vi "Configure DRAM Manager.vi"(0 "fpga interface in":refnum<k20>, 5 "serial output channels":string[](array[string]), 7 "elements per dram bank":u32, 9 "dram arbiter config":T1={"write grant time (clocks)"=1000, "read grant time (clocks)"=1000}, 11 "error in (no error)":errorcluster, 12 "write time slice":u16=500, 13 "request time slice":u16=500) -> (4 "fpga interface out":refnum<k20>, 6 "dram partition sizes (bytes)":u64[](array[numeric]), 15 "error out":errorcluster)   [LabVIEW 2023, in "GettingStarted_Gen_148X_Host.lvlib"]
uses:
  GettingStarted_Gen_148X_Host.lvlib
  Types/148x_Gen_FPGA_Reference.ctl
  <vilib>/Utility/error.llb/Error Cluster From Error Code.vi
  <vilib>/rvi/errors/niLvFpgaAdjustHostInterfaceError.vi
  <vilib>/rvi/interface/nirviReadWriteControl/nirviReadWriteControl.xnode
  <vilib>/rvi/interface/Simulation/niFpgaSimulationCallBeginRW.vi
  NiFpgaLv.dll
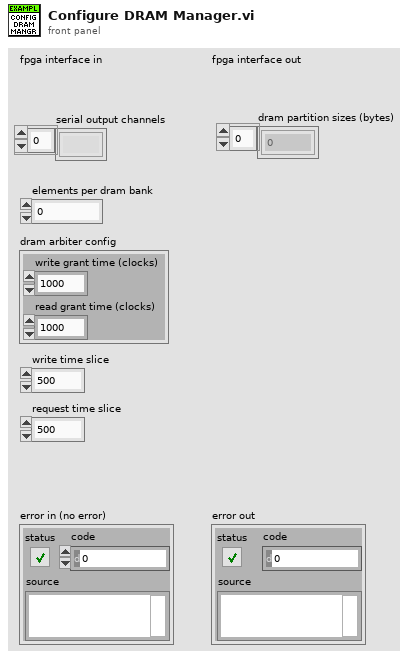
[diagram p1: front panel]
types:
  T1 = cluster{"write grant time (clocks)":u16, "read grant time (clocks)":u16}
  T2 = typedef "GettingStarted_Gen_148X_Host.lvlib/148x_Gen_FPGA_Reference.ctl" = refnum<k20>
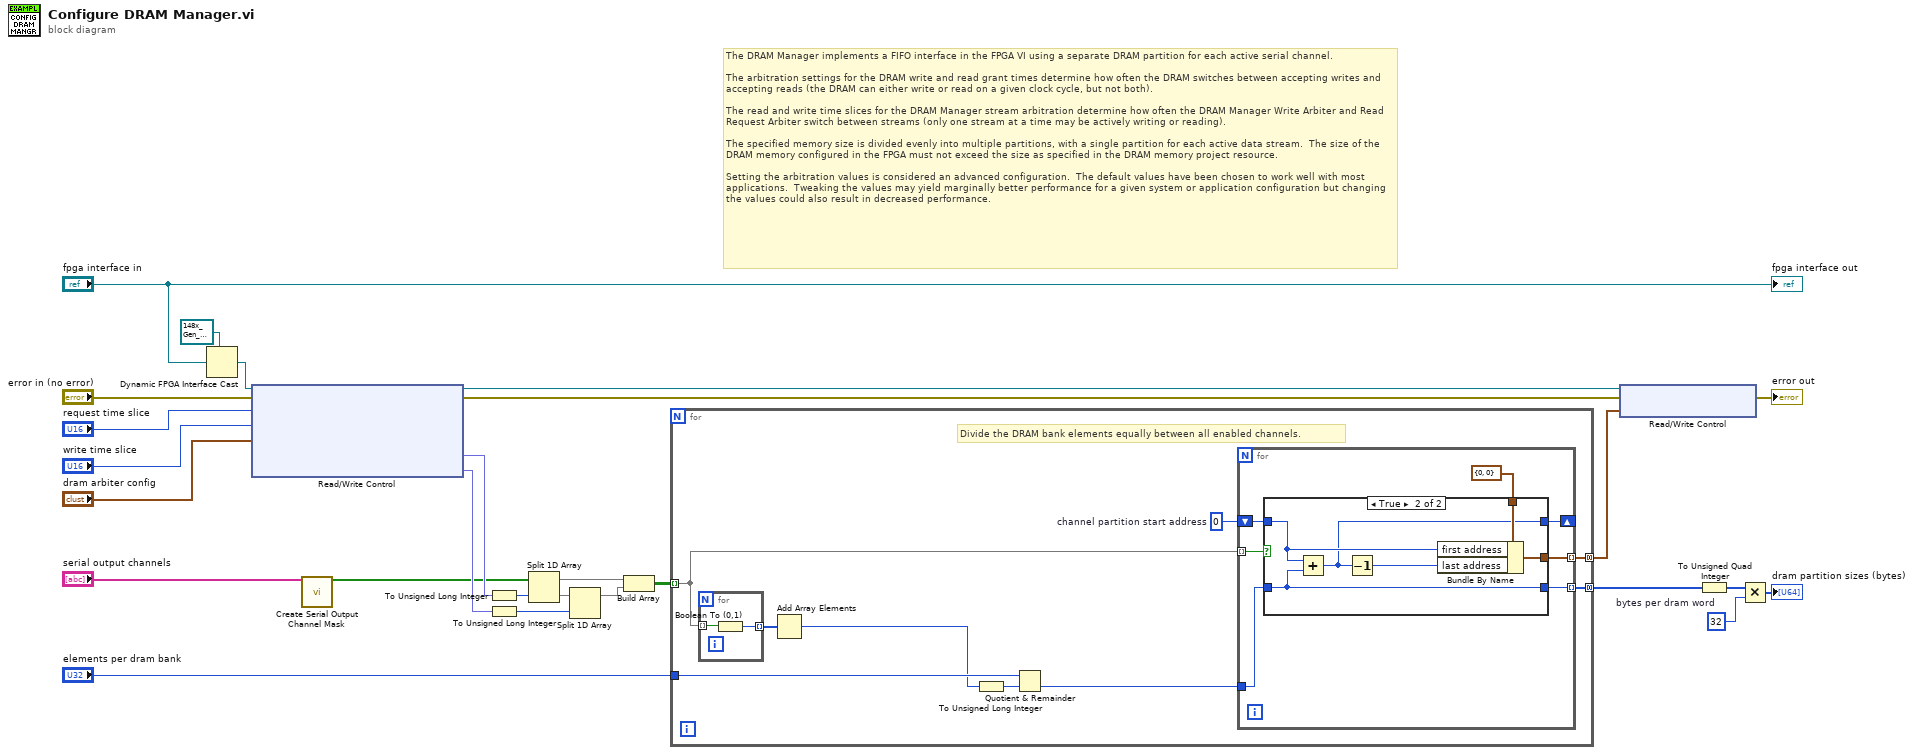
[diagram p0: block diagram]
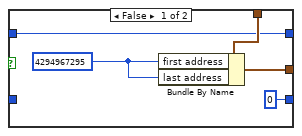
[diagram p2: hidden frame]
diagram:
  w4 = u64 32  # bytes per dram word
  # "The DRAM Manager implements a FIFO interface in the FPGA VI using a separate DRAM partition for each active serial channel.  \n\nThe arbitration settings for the DRAM write and read grant times determine how often the DRAM switches between accepting writes and accepting reads (the DRAM can either write or read on a given clock cycle, but not both).  \n\nThe read and write time slices for the DRAM Manager stream arbitration determine how often the DRAM Manager Write Arbiter and Read Request Arbiter switch between streams (only one stream at a time may be actively writing or reading).  \n\nThe specified memory size is divided evenly into multiple partitions, with a single partition for each active data stream.  The size of the DRAM memory configured in the FPGA must not exceed the size as specified in the DRAM memory project resource.  \n\nSetting the arbitration values is considered an advanced configuration.  The default values have been chosen to work well with most applications.  Tweaking the values may yield marginally better performance for a given system or application configuration but changing the values could also result in decreased performance."
  n1 = Dynamic FPGA Interface Cast(Session In=T2 refnum ("FPGA VI Reference Out"), Type="fpga interface in") -> (Session Out=w14:T2)
  n2 = xnode "Read/Write Control"("FPGA VI Reference In"=w14, "error in"="error in (no error)", "request time slice"="request time slice", "write time slice"="write time slice", "dram arbiter config"="dram arbiter config") -> ("FPGA VI Reference Out"=w22:T2, "error out"=w20:errorcluster, "dram manager 0.num active streams"=w19:fxp<+,3,3>, "dram manager 1.num active streams"=w8:fxp<+,3,3>)
  n3 = call "Create Serial Output Channel Mask.vi"("serial channels"="serial output channels") -> ("serial output channel mask"=w7:bool[])  [unwired: 14 in]
  n4 = To Unsigned Long Integer(number=w19) -> (unsigned 32bit integer=w10:u32)
  n5 = To Unsigned Long Integer(number=w8) -> (unsigned 32bit integer=w9:u32)
  n6 = Split 1D Array(array=w7, index=w10) -> (first subarray=w24:bool[], second subarray=w12:bool[])
  n7 = Split 1D Array(array=w12, index=w9) -> (first subarray=w11:bool[])  [unwired: 1 out]
  n8 = Build Array(w24, w11) -> (w23:bool[][])
  n9 = for {
    tunnel: "elements per dram bank" -> [w35]
    tunnel: w23 -> [w31] mode=indexing
    tunnel: [w28] -> w5 mode=concatenating
    tunnel: [w27] -> w2 mode=concatenating
    w30 = u32 0  # channel partition start address
    # "Divide the DRAM bank elements equally between all enabled channels."
    n10 = for {
      tunnel: w31 -> [w55] mode=indexing
      tunnel: [w54] -> w33 mode=indexing
      n11 = Boolean To (0,1)(Boolean=w55) -> (0, 1=w54:i16)
    }
    n12 = Add Array Elements(numeric array=w33) -> (sum=w32:i16)
    n13 = To Unsigned Long Integer(number=w32) -> (unsigned 32bit integer=w34:u32)
    n14 = Quotient & Remainder(x=w35, y=w34) -> (floor(x/y)=w29:u32)  [unwired: 1 out]
    n15 = for {
      tunnel: w31 -> [w42] mode=indexing
      shift-right: [w39] -> _
      shift-left: w30 -> [w41]
      tunnel: w29 -> [w40]
      tunnel: [w38] -> w28 mode=indexing
      tunnel: [w36] -> w27 mode=indexing
      n16 = case shown="True" w42 {
        tunnel: [w46 w52] -> w38
        tunnel: cluster{"first address":u32, "last address":u32} {"first address"=0, "last address"=0} ("si 0 dram partition config") -> [w45 w53]
        tunnel: w41 -> [w44 w51]
        tunnel: w40 -> [_ w48]
        tunnel: [w44 w50] -> w39
        tunnel: [u32 0 w48] -> w36
        frame False {
          w47 = u32 4294967295 ("partition first address")
          n17 = Bundle By Name(cluster=w45, "first address"=w47, "last address"=w47) -> (w46:cluster{"first address":u32, "last address":u32})
        }
        frame True {
          n18 = Add(x=w51, y=w48) -> (x+y=w50:u32)
          n19 = Decrement(x=w50) -> (x-1=w49:u32)
          n20 = Bundle By Name(cluster=w53, "first address"=w51, "last address"=w49) -> (w52:cluster{"first address":u32, "last address":u32})
        }
      }
    }
  }
  n21 = xnode "Read/Write Control"("FPGA VI Reference In"=w22, "error in"=w20, "dram partition configs"=w5) -> ("error out"=→"error out":errorcluster)  [unwired: 1 out]
  n22 = To Unsigned Quad Integer(1:w2) -> (0:w1:u64[])
  n23 = Multiply(x=w1, y=w4) -> (x*y=→"dram partition sizes (bytes)":u64[])
  "fpga interface out" <- "fpga interface in"
